vi "(SubVI) Start Record a Sine Wave Position.vi"(8 "error in (no error)":errorcluster, 9 "Axis (Enum)":enum16{"x", "y", "z"}(ring), 10 "Record time (s)":dbl, 11 "ADC rate (Hz)":dbl=20000.0) -> (0 "error out":errorcluster, 1 "Real Position Array (um)":dbl[](array[numeric]), 2 "Target Position Array (um)":dbl[](array[numeric]), 3 "Time Array (s)":dbl[](array[numeric]))   [LabVIEW 2014]
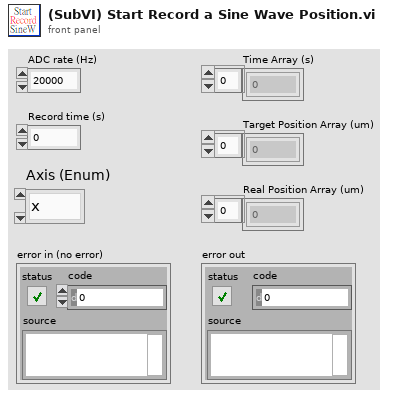
[diagram p1: front panel]
types:
  T1 = enum16{"Target position", "Current position", "position error"}
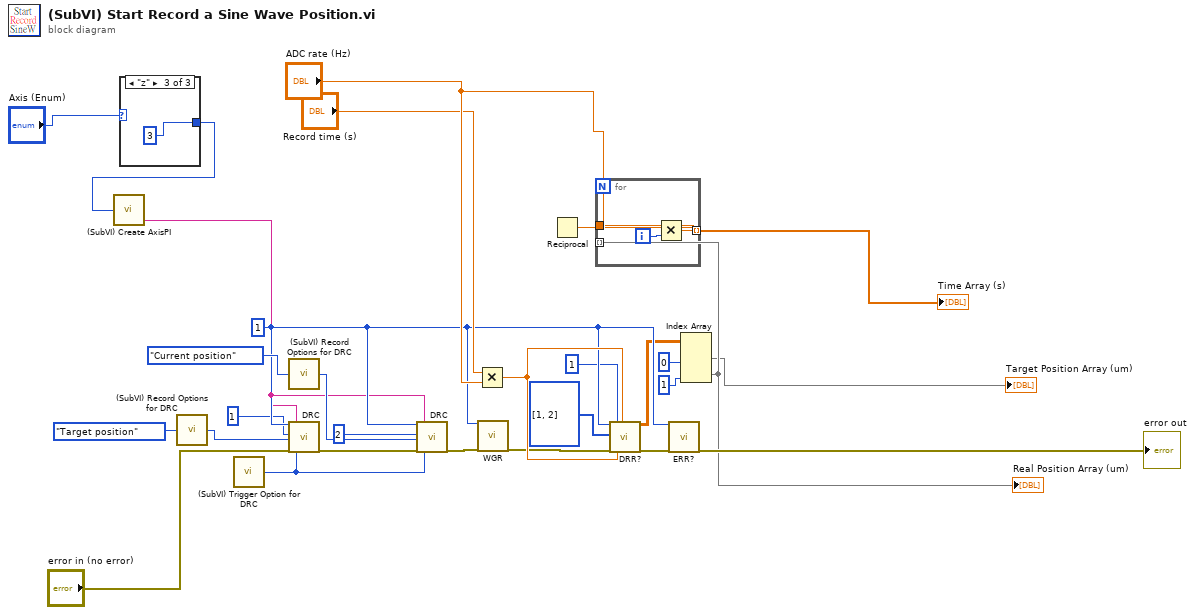
[diagram p0: block diagram]
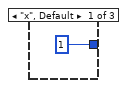
[diagram p2: hidden frame]
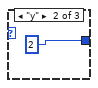
[diagram p3: hidden frame]
diagram:
  w14 = 1 ("System no.")
  n1 = case shown="\"z\"" "Axis (Enum)" {
    tunnel: [1 2 3] -> w1
    frame "x", Default {
    }
    frame "y" {
    }
    frame "z" {
    }
  }
  n2 = call "(SubVI) Create AxisPI.vi"("axis"=w1) -> ("Axis String"=w3:string)  [unwired: 2 in, 2 out]
  n3 = call "(SubVI) Record Options for DRC.vi"("Enum"=T1."Target position") -> ("Record options"=w18:i32)  [unwired: 4 in]
  n4 = call "(SubVI) Trigger Option for DRC.vi"() -> ("DRC trigger option"=w20:i32)  [unwired: 5 in]
  n5 = call "(SubVI) Record Options for DRC.vi"("Enum"=T1."Current position") -> ("Record options"=w19:i32)  [unwired: 4 in]
  n6 = call "DRC.vi"("System no."=w14, "Rec. table"=1 ("Numeric"), "Rec. option"=w18, "error in"="error in (no error)", "Source ID"=w3, "Trigger option"=w20) -> ("error out"=w9:errorcluster)  [unwired: 13 out]
  n7 = call "DRC.vi"("System no."=w14, "Rec. table"=2 ("Numeric"), "Rec. option"=w19, "error in"=w9, "Source ID"=w3, "Trigger option"=w20) -> ("error out"=w17:errorcluster)  [unwired: 13 out]
  n8 = Multiply(x="Record time (s)", y="ADC rate (Hz)") -> (x*y=w28:dbl)
  n9 = call "WGR.vi"("System no."=w14, "error in"=w17) -> ("error out"=w5:errorcluster)  [unwired: 2 in, 15 out]
  n10 = Reciprocal(x="ADC rate (Hz)") -> (1/x=w22:dbl)
  n11 = call "DRR?.vi"("System no."=w14, "Rec. table IDs"=i32[] [1, 2], "error in"=w5, "Xo"=1, "N"=w28, "Nmax"=w28) -> ("Data"=w12:dbl[][], "error out"=w4:errorcluster)  [unwired: 2 in, 10 out]
  n12 = call "ERR?.vi"("System no."=w14, "error in"=w4) -> ("error out"=→"error out":errorcluster)  [unwired: 17 out]
  n13 = Index Array(array=w12, index (col) #1=0 ("Disabled Index (col)"), index (col) #2=1 ("Disabled Index (col)")) -> (element #1=→"Target Position Array (um)":dbl[], element #2=w25:dbl[])  [unwired: 2 in]
  "Real Position Array (um)" <- w25
  n14 = for {
    tunnel: w25 -> [_] mode=indexing
    tunnel: w22 -> [w34]
    tunnel: [w33] -> w23 mode=indexing
    i -> [w35]
    n15 = Multiply(x=w34, y=w35) -> (x*y=w33:dbl)
  }
  "Time Array (s)" <- w23
